vi "DataLog Database Infos_srv.vi"(0 "method":T9, 1 "initial number (NaN)":dbl=nan format="%.2f", 2 "tag index/change#":i32, 5 "tag or base tag":string, 7 "tag config in":T4 {"logging parameters" format="%.2e"; "precision" items=["0", "1", "2", "3", "4", "5", "6", "7", "8", "9", "10", "11", "12", "13", "14", "15", "16", "17"]; "limit delay" format="%.2e"; "deadband" format="%.2e"}, 9 "subsets in":T1[](array[typedef]), 11 "meta specifier (not a meta)":T3=enum."not a meta", 12 "certificate in":string, 13 "initial string (\"\")":string, 14 "database (current)":string) -> (3 "mode":T2, 4 "tag config list":T4[](array[typedef]) {"logging parameters" format="%.2e"; "precision" items=["0", "1", "2", "3", "4", "5", "6", "7", "8", "9", "10", "11", "12", "13", "14", "15", "16", "17"]; "limit delay" format="%.2e"; "deadband" format="%.2e"}, 6 "#tags/change#":i32, 8 "tag config out":T4 {"logging parameters" format="%.2e"; "precision" items=["0", "1", "2", "3", "4", "5", "6", "7", "8", "9", "10", "11", "12", "13", "14", "15", "16", "17"]; "limit delay" format="%.2e"; "deadband" format="%.2e"}, 10 "subsets out":T1[](array[typedef]), 15 "error out":errorcluster)   [LabVIEW 2012]
doc: "Security and remote calling wrapper around the database info object instances."
uses:
  typedefs/t_DataLog Tag Info List Methods.ctl
  typedefs/t_Datalog Datebase Modes.ctl
  typedefs/clusters/t_DataLog Tag Config.ctl
  typedefs/t_DataLog Temporal Types.ctl
  typedefs/t_DataLog Value Types.ctl
  typedefs/t_DataLog Numerical Format.ctl
  typedefs/t_DataLog Logging Algorithms.ctl
  typedefs/clusters/t_DataLog Tag Subset.ctl
  typedefs/et_DataLog Meta Tag Specifier.ctl
  typedefs/t_DataLog Databases Methods.ctl
  clientsrv/typedefs/t_ClientSrv Access Levels.ctl
panel:
  # "Update panel typedef\nafter changing panel."
  # "Update panel typedef\nafter changing panel."
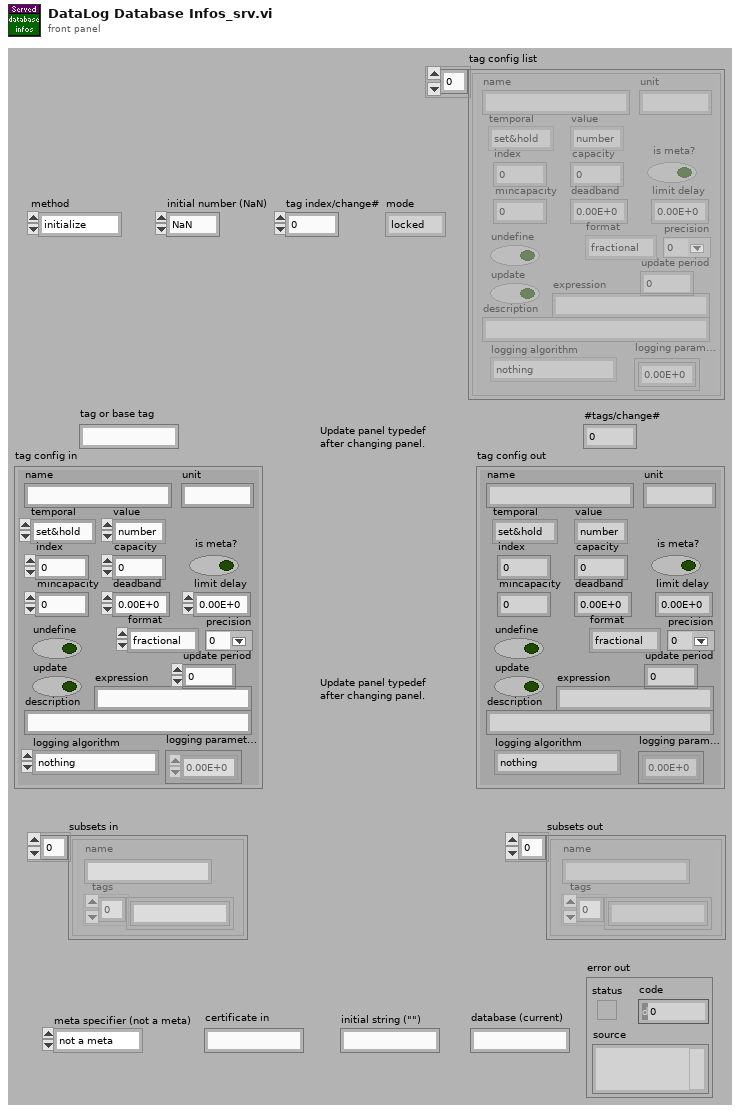
[diagram p1: front panel]
types:
  T1 = typedef "t_DataLog Tag Subset.ctl" = cluster{"name":string, "tags":string[]}
  T2 = typedef "t_Datalog Datebase Modes.ctl" = enum16{"locked", "unlocked", "live", "mirrored"}
  T3 = typedef "et_DataLog Meta Tag Specifier.ctl" = enum32{"warn_lo", "warn_hi", "A_lo", "A_hi", "B_lo", "B_hi", "C_lo", "C_hi", "D_lo", "D_hi", "E_lo", "E_hi", "F_lo", "F_hi", "G_lo", "G_hi", "H_lo", "H_hi", "I_lo", "I_hi", "J_lo", "J_hi", "K_lo", "K_hi", "L_lo", "L_hi", "M_lo", "M_hi", "N_lo", "N_hi", "min", "max", "not a meta"}
  T4 = typedef "t_DataLog Tag Config.ctl" = cluster{"name":string, "unit":string, "temporal":T5, "value":T6, "index":i32, "capacity":i32, "is meta?":bool, "mincapacity":i32, "deadband":dbl, "limit delay":dbl, "format":T7, "precision":u8, "undefine":bool, "update":bool, "update period":u16, "expression":string, "description":string, "logging algorithm":T8, "logging parameters":dbl[]}
  T5 = typedef "t_DataLog Temporal Types.ctl" = enum16{"set&hold", "sample", "event"}
  T6 = typedef "t_DataLog Value Types.ctl" = enum16{"number", "string"}
  T7 = typedef "t_DataLog Numerical Format.ctl" = enum8{"fractional", "exponential", "engineering"}
  T8 = typedef "t_DataLog Logging Algorithms.ctl" = enum16{"nothing", "changes", "everything", "every Nth", "time threshold", "value threshold + prior", "t or v threshold", "t or v threshold + prior"}
  T9 = typedef "t_DataLog Tag Info List Methods.ctl" = enum16{"initialize", "create", "create empty", "rename", "delete", "test tag", "get", "get by name", "get default", "get list", "get path", "get subsets", "set subsets", "set config", "set capacity", "#tags", "go live", "set unlocked", "set mirrored"}
  T10 = typedef "t_DataLog Databases Methods.ctl" = enum16{"initialize", "get ref", "get names", "cleanup"}
  T11 = typedef "t_ClientSrv Access Levels.ctl" = enum16{"observer", "operator", "local"}
  T12 = typedef "t_DataLog Database Info Pane.ctl" = refnum<vi>
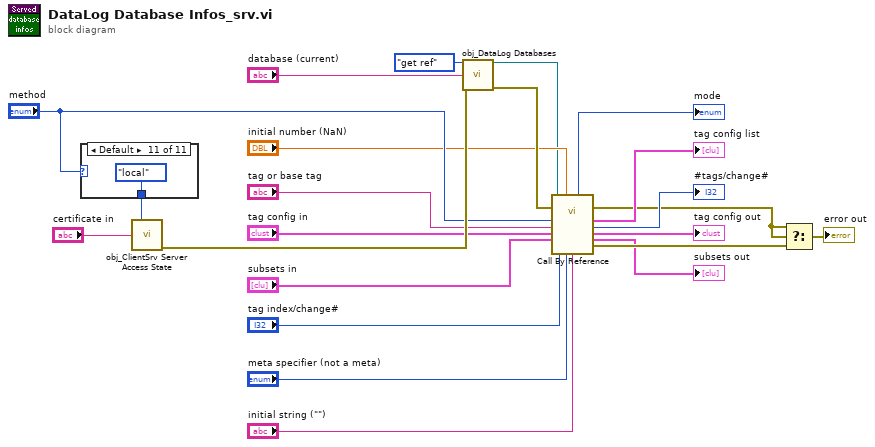
[diagram p0: block diagram]
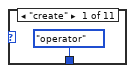
[diagram p2: hidden frame]
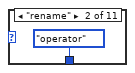
[diagram p3: hidden frame]
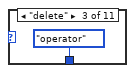
[diagram p4: hidden frame]
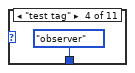
[diagram p5: hidden frame]
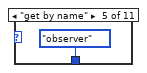
[diagram p6: hidden frame]
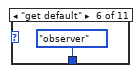
[diagram p7: hidden frame]
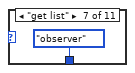
[diagram p8: hidden frame]
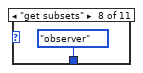
[diagram p9: hidden frame]
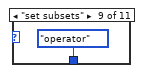
[diagram p10: hidden frame]
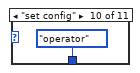
[diagram p11: hidden frame]
diagram:
  n1 = case shown="Default" "method" {
    tunnel: [t_ClientSrv_Access_Levels."operator" ("access level") t_ClientSrv_Access_Levels."operator" ("access level") t_ClientSrv_Access_Levels."operator" ("access level") t_ClientSrv_Access_Levels."observer" ("access level") t_ClientSrv_Access_Levels."observer" ("access level") t_ClientSrv_Access_Levels."observer" ("access level") t_ClientSrv_Access_Levels."observer" ("access level") t_ClientSrv_Access_Levels."observer" ("access level") t_ClientSrv_Access_Levels."operator" ("access level") t_ClientSrv_Access_Levels."operator" ("access level") t_ClientSrv_Access_Levels."local" ("access level")] -> w23
    frame "create" {
    }
    frame "rename" {
    }
    frame "delete" {
    }
    frame "test tag" {
    }
    frame "get by name" {
    }
    frame "get default" {
    }
    frame "get list" {
    }
    frame "get subsets" {
    }
    frame "set subsets" {
    }
    frame "set config" {
    }
    frame Default {
    }
  }
  n2 = call "obj_ClientSrv Server Access State.vi"("access level"=w23, "certificate in"="certificate in") -> ("error out"=w19:errorcluster)  [unwired: 11 in, 2 out]
  n3 = call "obj_DataLog Databases.vi"("method"=t_DataLog_Databases_Methods."get ref", "database (current)"="database (current)", "error in (no error)"=w19) -> ("database ref"=w5:T12, "error out"=w20:errorcluster)  [unwired: 10 in, 1 out]
  n4 = call-by-ref "?"(reference=w5, error in=w20, "method"="method", "initial number (NaN)"="initial number (NaN)", "tag or base tag"="tag or base tag", "tag config in"="tag config in", "subsets in"="subsets in", "tag index/change#"="tag index/change#", "meta specifier (not a meta)"="meta specifier (not a meta)", "initial string (\"\")"="initial string (\"\")") -> (error out=w6:errorcluster, "mode"=→"mode":T2, "tag config list"=→"tag config list":T4[], "#tags/change#"=→"#tags/change#":i32, "tag config out"=→"tag config out":T4, "subsets out"=→"subsets out":T1[], 15:"error out"=w7:errorcluster)  [unwired: 1 in, 2 out]
  n5 = Select(t=w6, s=w6, f=w7) -> (s? t:f=→"error out":errorcluster)
